vi "Circular Buffer(1D Wfm with Attributes).vi"(7 "Buffer Size":T3, 8 "error in (no error)":errorcluster, 9 "Read Size":i32, 10 "Operation":T1, 11 "Data In":waveform(dbl)) -> (0 "error out":errorcluster, 1 "Elements Remaining":i32, 2 "Buffer Status":T2, 3 "Data Out":waveform(dbl))   [LabVIEW 2016, in "Circular Buffer.lvlib"]
doc: "This VI implements a circular buffer which data can be written to and read from. There can only be one buffer per data type at once, but you can have multiple buffers of different types at the same time. For example, you can have a buffer of Wfm data types as well as I32s in the same VI. You cannot have two independent buffers of I32s."
uses:
  Circular Buffer.lvlib
  Controls/Circular Buffer Status.ctl
  Controls/Circular Buffer Operations.ctl
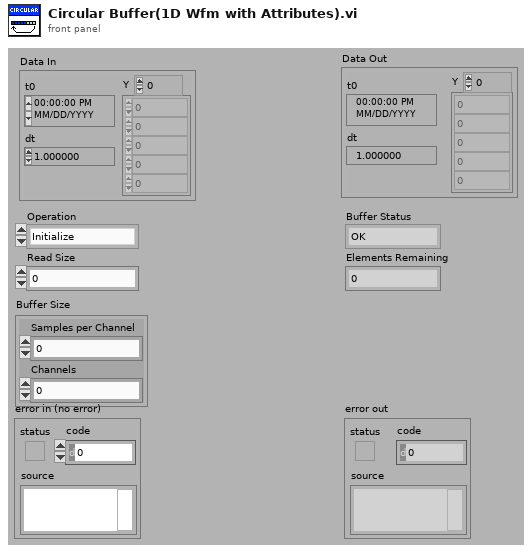
[diagram p1: front panel]
types:
  T1 = typedef "Circular Buffer.lvlib/Circular Buffer Operations.ctl" = enum16{"Initialize", "Get Backlog", "Write", "Read (continuous)", "Read (most recent)"}
  T2 = typedef "Circular Buffer.lvlib/Circular Buffer Status.ctl" = enum16{"OK", "Overflow", "Underflow"}
  T3 = cluster{"Samples per Channel":u32, "Channels":u32}
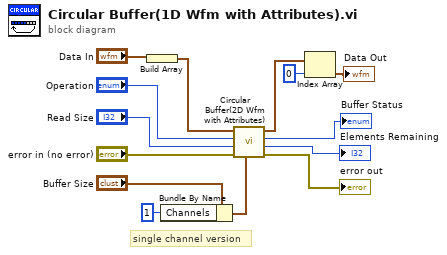
[diagram p0: block diagram]
diagram:
  # "single channel version"
  n1 = Build Array("Data In") -> (w10:waveform(dbl)[])
  n2 = Bundle By Name(cluster="Buffer Size", "Channels"=1) -> (w1:T3)
  n3 = call "Circular Buffer(2D Wfm with Attributes).vi"("Buffer Size"=w1, "error in (no error)"="error in (no error)", "Read Size"="Read Size", "Operation"="Operation", "Data In"=w10) -> ("error out"=→"error out":errorcluster, "Elements Remaining"=→"Elements Remaining":i32, "Buffer Status"=→"Buffer Status":T2, "Data Out"=w6:waveform(dbl)[])  [unwired: 1 in, 2 out]
  n4 = Index Array(array=w6, index=0) -> (element=→"Data Out":waveform(dbl))
